vi "Send Packet.vi"(6 "error in (no error) 2":errorcluster, 7 "?":T2, 8 "Log string 2":string, 9 "SerialPortRef 2":T1) -> (0 "error out 2":errorcluster, 3 "SerialPortRef out 2":T1)   [LabVIEW 2015]
uses:
  <vilib>/Rock Robotics/WPI/SerialPort/WPI_SerialPortRef.ctl
  Old code/packet types.ctl
panel:
  in  "?":T2
  out "Sent string":string
  out "error out":errorcluster
  in  "error in (no error)":errorcluster
  out "SerialPortRef out":T1
  in  "SerialPortRef":T1
  in  "Log string":string
  # "Type:"
  # "Cannot contain line breaks or the character 0x00"
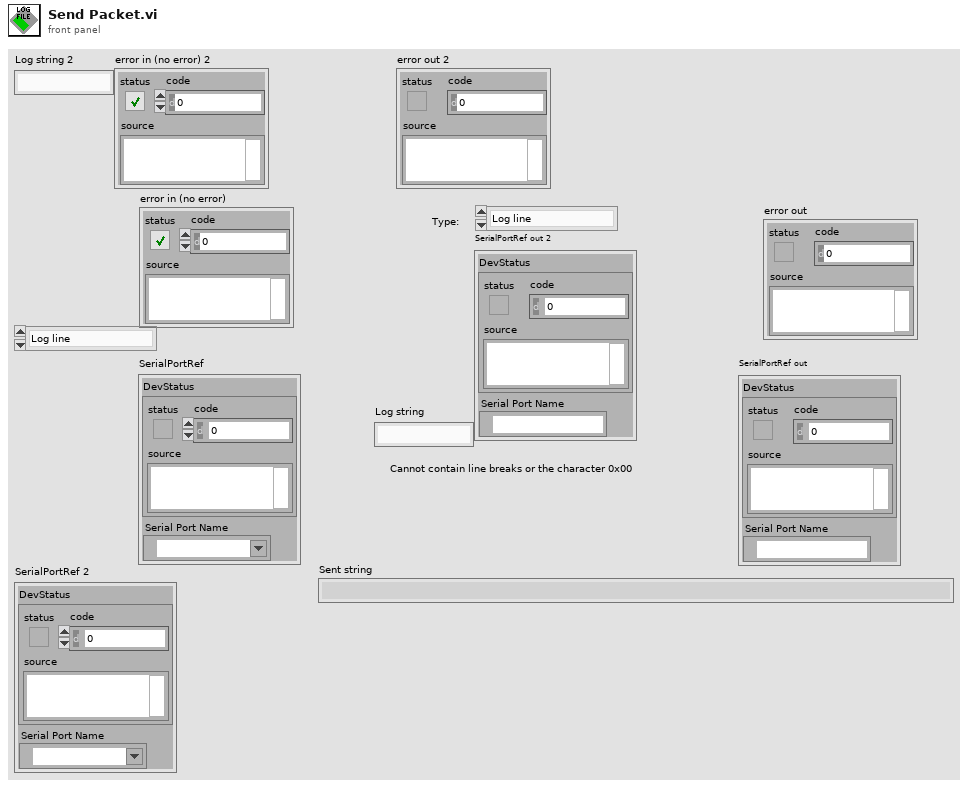
[diagram p1: front panel]
types:
  T1 = typedef "WPI_SerialPortRef.ctl" = cluster{"DevStatus":errorcluster, "Serial Port Name":refnum<visa-resource-name>}
  T2 = typedef "packet types.ctl" = enum16{"Log line", "Open File", "Close File", "Send Header", "Set Time", "Send to LCD"}
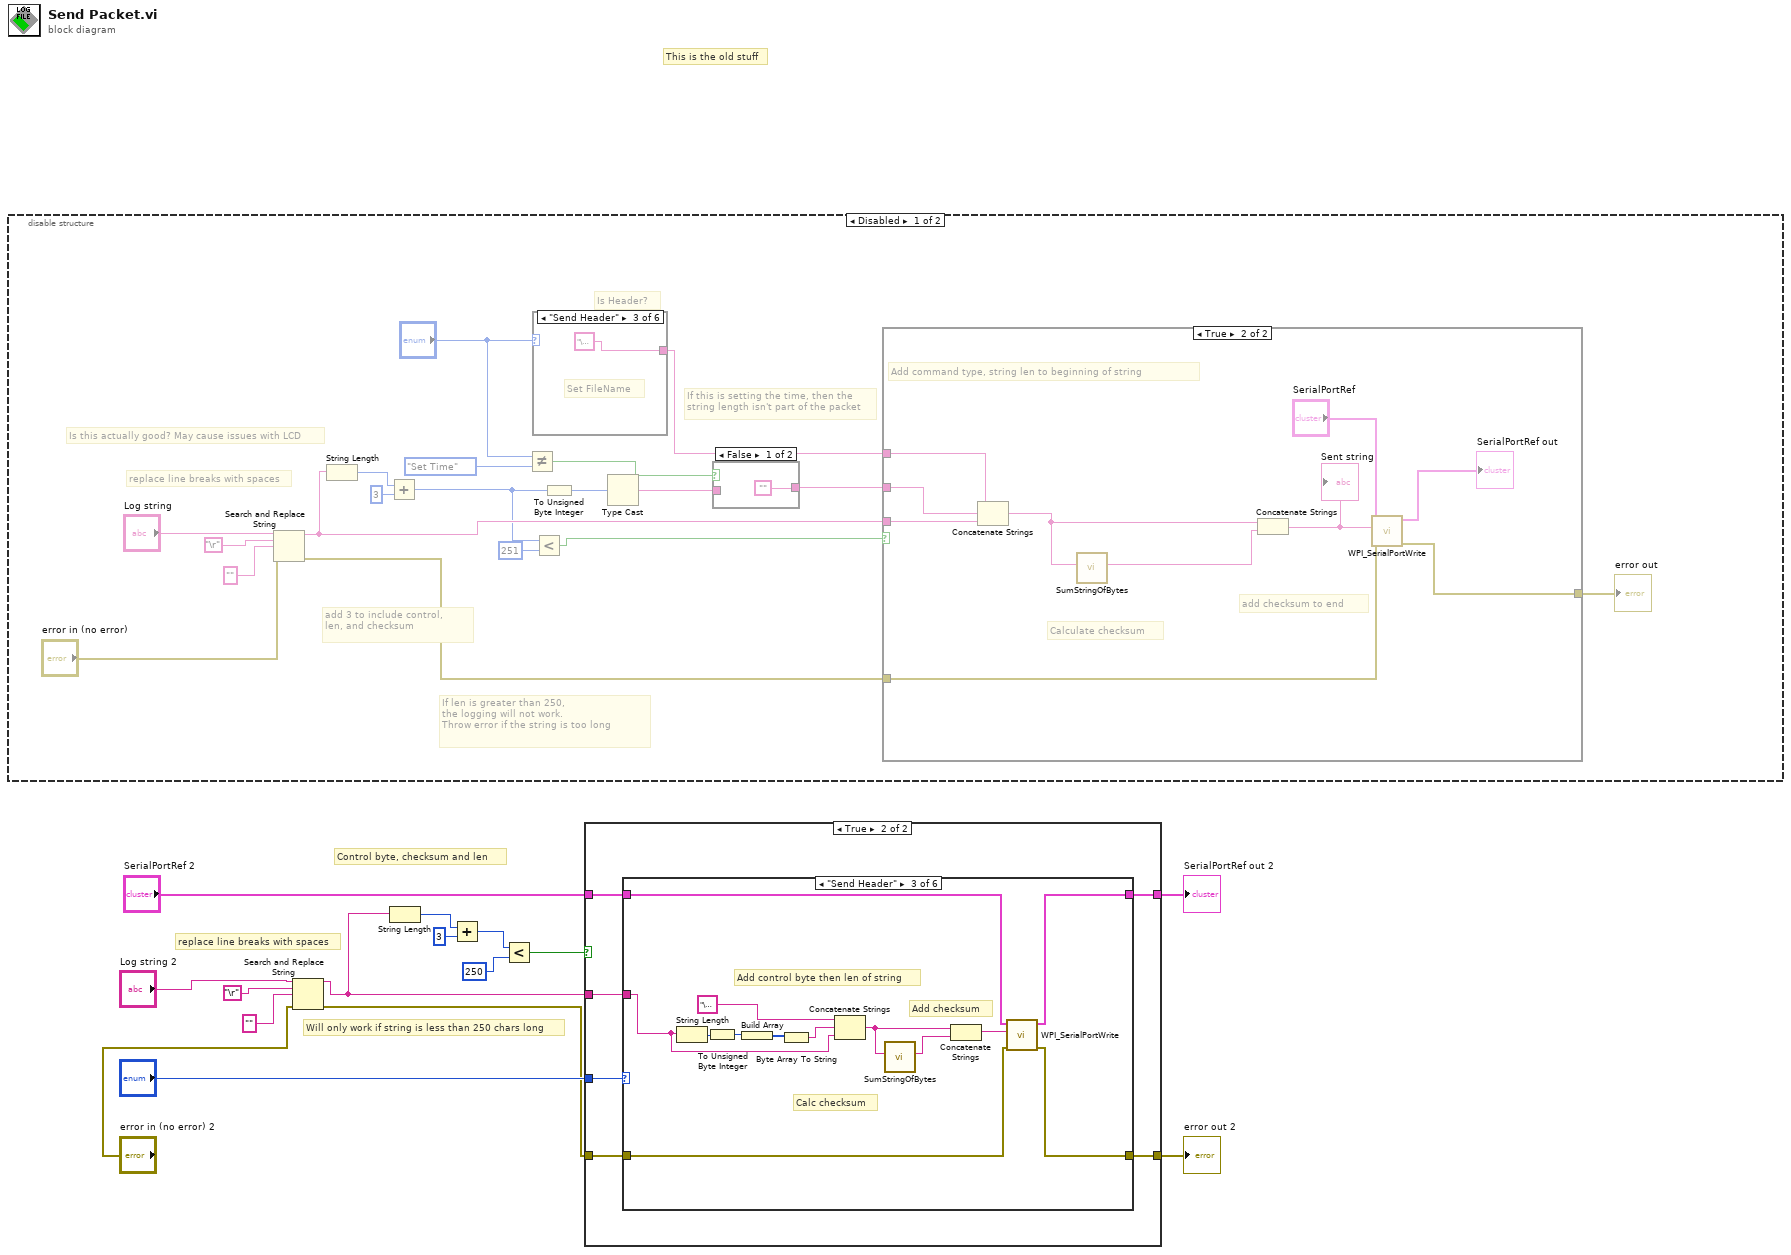
[diagram p0: block diagram]
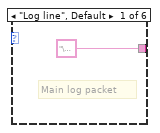
[diagram p3: hidden frame]
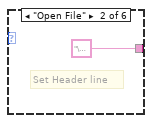
[diagram p4: hidden frame]
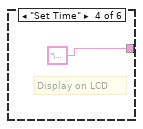
[diagram p5: hidden frame]
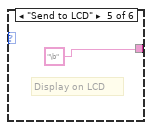
[diagram p6: hidden frame]
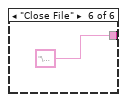
[diagram p7: hidden frame]
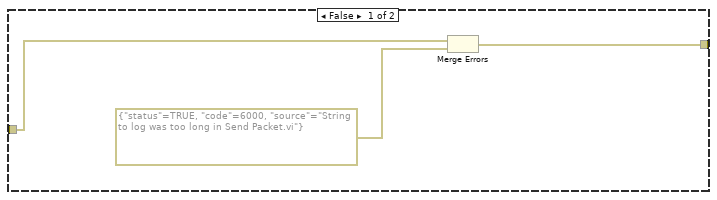
[diagram p8: hidden frame]
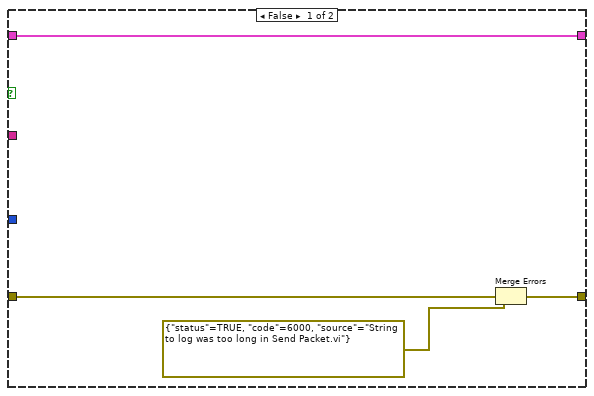
[diagram p10: hidden frame]
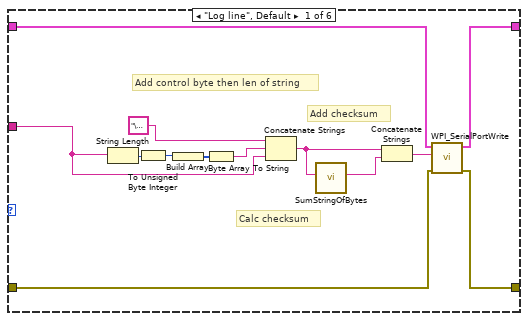
[diagram p11: hidden frame]
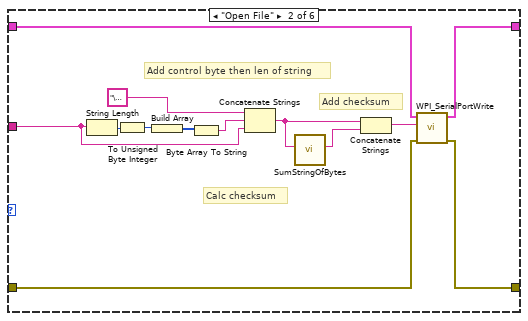
[diagram p12: hidden frame]
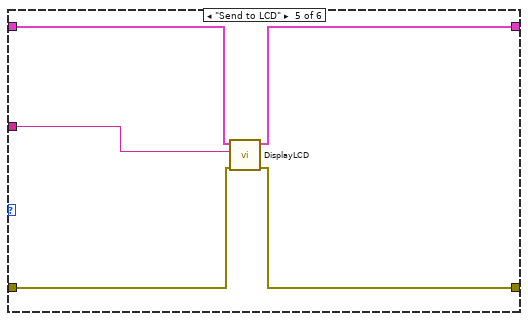
[diagram p14: hidden frame]
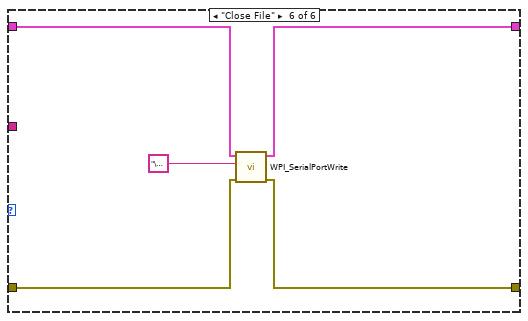
[diagram p15: hidden frame]
diagram:
  # "This is the old stuff"
  # "Control byte, checksum and len"
  # "Will only work if string is less than 250 chars long"
  # "replace line breaks with spaces"
  n1 = disable-structure shown="Disabled" {
    frame Disabled {
      # "If this is setting the time, then the \nstring length isn't part of the packet"
      # "Is this actually good? May cause issues with LCD"
      # "Is Header?"
      # "If len is greater than 250,\nthe logging will not work.\nThrow error if the string is too long"
      # "add 3 to include control, \nlen, and checksum"
      # "replace line breaks with spaces"
      n2 = Search and Replace String(input string="Log string", search string="\r", replace string="" ("replace string (\"\")"), error in="error in (no error)") -> (result string=w27:string, error out=w30:errorcluster)  [unwired: 4 in, 2 out]
      n3 = String Length(string=w27) -> (length=w29:i32)
      n4 = Add(x=w29, y=3) -> (x+y=w21:i32)
      n5 = Not Equal?(x="?", y=packet_types."Set Time") -> (x != y?=w16:bool)
      n6 = case shown="\"Send Header\"" "?" {
        tunnel: ["\u0001" ("string") "\u0003" ("string") "\u0002" ("string") "\u0005" ("string") "\b" ("string") "\u0004" ("string")] -> w23
        frame "Log line", Default {
          # "Main log packet"
        }
        frame "Open File" {
          # "Set Header line"
        }
        frame "Send Header" {
          # "Set FileName"
        }
        frame "Set Time" {
          # "Display on LCD"
        }
        frame "Send to LCD" {
          # "Display on LCD"
        }
        frame "Close File" {
        }
      }
      n7 = Less?(x=w21, y=251) -> (x < y?=w24:bool)
      n8 = To Unsigned Byte Integer(number=w21) -> (unsigned 8bit integer=w22:u8)
      n9 = Type Cast(x=w22) -> (*(type *) &x=w20:string)  [unwired: 1 in]
      n10 = case shown="False" w16 {
        tunnel: w20 -> [_ w36]
        tunnel: ["" w36] -> w19
        frame False {
        }
        frame True {
        }
      }
      n11 = case shown="True" w24 {
        tunnel: w30 -> [w45 w53]
        tunnel: w23 -> [_ w52]
        tunnel: w19 -> [_ w46]
        tunnel: w27 -> [_ w48]
        tunnel: [w43 w47] -> w26
        frame False {
          n12 = Merge Errors(w45, errorcluster {"status"=TRUE, "code"=6000, "source"="String to log was too long in Send Packet.vi"} ("error out")) -> (w43:errorcluster)
        }
        frame True {
          # "add checksum to end"
          # "Add command type, string len to beginning of string"
          # "Calculate checksum"
          n13 = Concatenate Strings(w52, w46, w48) -> (w51:string)
          n14 = call "SumStringOfBytes.vi"("String Of Bytes"=w51) -> ("SumAsString"=w50:string)  [unwired: 10 in]
          n15 = Concatenate Strings(w51, w50) -> (w49:string)
          "Sent string" <- w49
          n16 = call <vilib>:"WPI_SerialPortWrite.vi"("error in (no error)"=w53, "Buffer"=w49, "SerialPortRef"="SerialPortRef") -> ("error out"=w47:errorcluster, "SerialPortRef"=→"SerialPortRef out":T1)  [unwired: 6 in, 1 out]
        }
      }
      "error out" <- w26
    }
    frame Enabled {
    }
  }
  n17 = Search and Replace String(input string="Log string 2", search string="\r", replace string="" ("replace string (\"\")"), error in="error in (no error) 2") -> (result string=w4:string, error out=w1:errorcluster)  [unwired: 4 in, 2 out]
  n18 = String Length(string=w4) -> (length=w8:i32)
  n19 = Add(x=w8, y=3) -> (x+y=w6:i32)
  n20 = Less?(x=w6, y=250) -> (x < y?=w3:bool)
  n21 = case shown="True" w3 {
    tunnel: "?" -> [_ w65]
    tunnel: "SerialPortRef 2" -> [w56 w64]
    tunnel: w1 -> [w58 w63]
    tunnel: w4 -> [_ w62]
    tunnel: [w56 w61] -> w10
    tunnel: [w57 w60] -> w9
    frame False {
      n22 = Merge Errors(w58, errorcluster {"status"=TRUE, "code"=6000, "source"="String to log was too long in Send Packet.vi"} ("error out")) -> (w57:errorcluster)
    }
    frame True {
      n23 = case shown="\"Send Header\"" w65 {
        tunnel: w63 -> [w70 w82 w94 w105 w109 w113]
        tunnel: w64 -> [w71 w83 w96 w106 w111 w115]
        tunnel: w62 -> [w74 w84 w92 _ w107 _]
        tunnel: [w68 w81 w95 w106 w110 w114] -> w61
        tunnel: [w69 w80 w93 w105 w108 w112] -> w60
        frame "Log line", Default {
          # "Add checksum"
          # "Add control byte then len of string"
          # "Calc checksum"
          n24 = String Length(string=w74) -> (length=w67:i32)
          n25 = To Unsigned Byte Integer(number=w67) -> (unsigned 8bit integer=w66:u8)
          n26 = Build Array(w66) -> (w78:u8[])
          n27 = Byte Array To String(unsigned byte array=w78) -> (string=w77:string)
          n28 = Concatenate Strings("\u0001", w77, w74) -> (w73:string)
          n29 = call "SumStringOfBytes.vi"("String Of Bytes"=w73) -> ("SumAsString"=w75:string)  [unwired: 10 in]
          n30 = Concatenate Strings(w73, w75) -> (w72:string)
          n31 = call <vilib>:"WPI_SerialPortWrite.vi"("error in (no error)"=w70, "Buffer"=w72, "SerialPortRef"=w71) -> ("error out"=w69:errorcluster, "SerialPortRef"=w68:T1)  [unwired: 6 in, 1 out]
        }
        frame "Open File" {
          # "Calc checksum"
          # "Add checksum"
          # "Add control byte then len of string"
          n32 = String Length(string=w84) -> (length=w85:i32)
          n33 = To Unsigned Byte Integer(number=w85) -> (unsigned 8bit integer=w88:u8)
          n34 = Build Array(w88) -> (w87:u8[])
          n35 = Byte Array To String(unsigned byte array=w87) -> (string=w86:string)
          n36 = Concatenate Strings("\u0003", w86, w84) -> (w90:string)
          n37 = call "SumStringOfBytes.vi"("String Of Bytes"=w90) -> ("SumAsString"=w91:string)  [unwired: 10 in]
          n38 = Concatenate Strings(w90, w91) -> (w79:string)
          n39 = call <vilib>:"WPI_SerialPortWrite.vi"("error in (no error)"=w82, "Buffer"=w79, "SerialPortRef"=w83) -> ("error out"=w80:errorcluster, "SerialPortRef"=w81:T1)  [unwired: 6 in, 1 out]
        }
        frame "Send Header" {
          # "Calc checksum"
          # "Add checksum"
          # "Add control byte then len of string"
          n40 = String Length(string=w92) -> (length=w103:i32)
          n41 = To Unsigned Byte Integer(number=w103) -> (unsigned 8bit integer=w100:u8)
          n42 = Build Array(w100) -> (w101:u8[])
          n43 = Byte Array To String(unsigned byte array=w101) -> (string=w102:string)
          n44 = Concatenate Strings("\u0002", w102, w92) -> (w98:string)
          n45 = call "SumStringOfBytes.vi"("String Of Bytes"=w98) -> ("SumAsString"=w97:string)  [unwired: 10 in]
          n46 = Concatenate Strings(w98, w97) -> (w104:string)
          n47 = call <vilib>:"WPI_SerialPortWrite.vi"("error in (no error)"=w94, "Buffer"=w104, "SerialPortRef"=w96) -> ("error out"=w93:errorcluster, "SerialPortRef"=w95:T1)  [unwired: 6 in, 1 out]
        }
        frame "Set Time" {
        }
        frame "Send to LCD" {
          n48 = call "DisplayLCD.vi"("error in (no error)"=w109, "Display string"=w107, "SerialPortRef"=w111) -> ("error out"=w108:errorcluster, "SerialPortRef 2"=w110:T1)  [unwired: 7 in]
        }
        frame "Close File" {
          n49 = call <vilib>:"WPI_SerialPortWrite.vi"("error in (no error)"=w113, "Buffer"="\u0004", "SerialPortRef"=w115) -> ("error out"=w112:errorcluster, "SerialPortRef"=w114:T1)  [unwired: 6 in, 1 out]
        }
      }
    }
  }
  "SerialPortRef out 2" <- w10
  "error out 2" <- w9
